vi "P4CMD Dialog - File Properties.vi"(7 "fstat data":string, 8 "error in (no error)":errorcluster, 10 "opened data":string, 11 "source control reference in":T1) -> (0 "error out":errorcluster)   [LabVIEW 2017, in "NI_SCC_P4CMD.lvlib"]
uses:
  <vilib>/SourceControl/Providers/P4CMD/NI_SCC_P4CMD.lvlib
  <vilib>/SourceControl/sccapi/SCCAPI Refnum.ctl
  <vilib>/SourceControl/Providers/P4CMD/P4CMD Operations.ctl
  <vilib>/event_ctls.llb/eventvkey.ctl
  <vilib>/SourceControl/sccapi/NI_SCC.lvlib
panel:
  in  "Describe":bool
  in  "help":bool
  out "locked by":string caption="Locked By:"
  in  "opened by":i32(listbox) caption="Opened For:"
  out "last mode time":string caption="Last ModTime:"
  out "head change":string caption="Head Change:"
  out "have revision":string caption="Have Revision:"
  out "head action":string caption="Head Action:"
  out "head revision":string caption="Head Revision:"
  out "file type":string caption="File Type:"
  out "client path":string caption="Client Path:"
  out "depot path":string caption="Depot Path:"
  in  "ok":bool
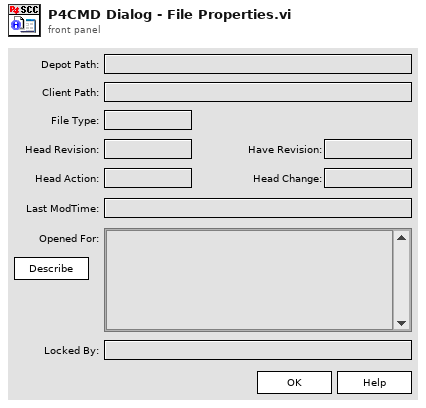
[diagram p1: front panel]
types:
  T1 = typedef "NI_SCC.lvlib/SCCAPI Refnum.ctl" = refnum<k1>
  T2 = typedef "NI_SCC_P4CMD.lvlib/P4CMD Operations.ctl" = enum16{"get all clients", "get all users", "describe changelist", "sync from depot", "open for edit", "submit to depot", "revert", "add to depot", "remove from depot", "print files revisions", "compare client file", "print depot file contents", "list opened files", "get file info", "lock files", "edit changelist spec", "info", "set variables"}
  T3 = typedef "eventvkey.ctl" = enum16{"ASCII", "Enter", "Return", "Shift", "Ctrl", "Alt", "Cmd", "Opt", "Caps", "NumLock", "Clear", "Break", "Up", "Down", "Left", "Right", "Insert", "Delete", "Home", "End", "PageUp", "PageDown", "Escape", "Help", "Pause", "ScrollLock", "F1", "F2", "F3", "F4", "F5", "F6", "F7", "F8", "F9", "F10", "F11", "F12", "F13", "F14", "F15", "F16", "F17", "F18", "F19", "F20", "F21", "F22", "F23", "F24", "Play", "VolumeUp", "VolumeDown", "Mute", "Two Byte Char"}
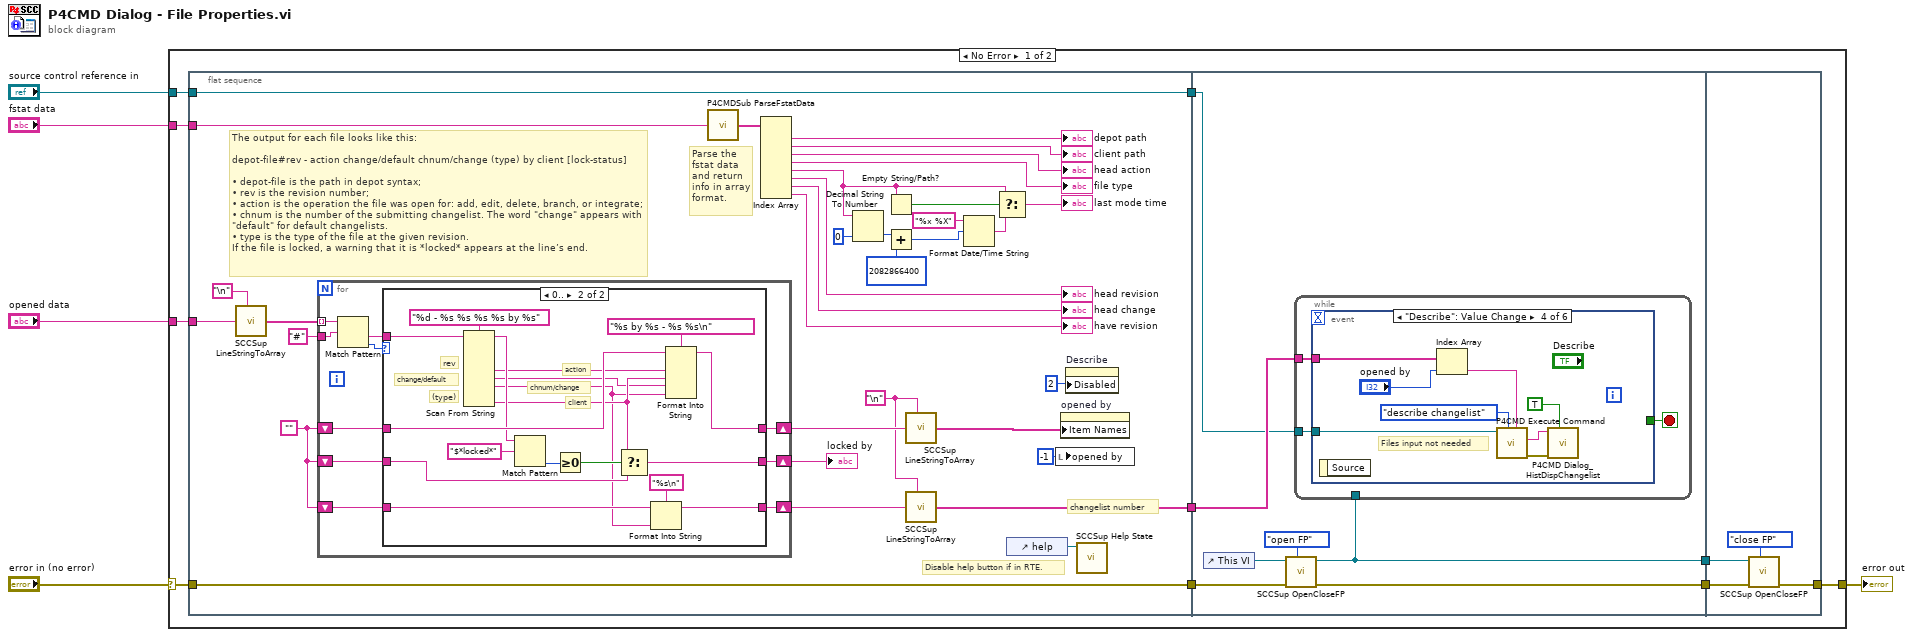
[diagram p0: block diagram]
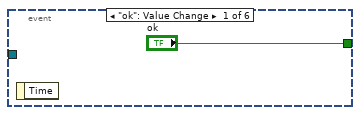
[diagram p3: hidden frame]
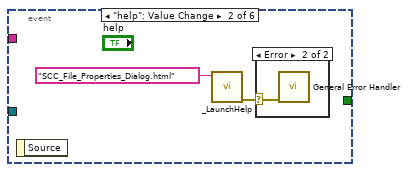
[diagram p4: hidden frame]
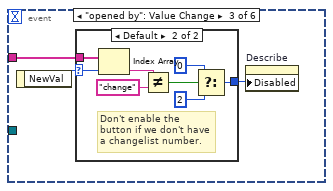
[diagram p6: hidden frame]
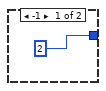
[diagram p7: hidden frame]
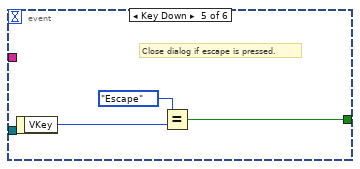
[diagram p8: hidden frame]
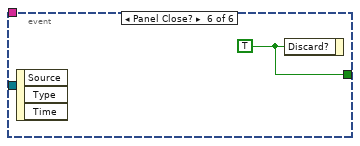
[diagram p9: hidden frame]
diagram:
  n1 = case shown="No Error" "error in (no error)" {
    selector: "error in (no error)" -> [w15 w123]
    tunnel: [w11 w123] -> w4
    tunnel: "fstat data" -> [w10 _]
    tunnel: "opened data" -> [w9 _]
    tunnel: "source control reference in" -> [w7 _]
    frame No Error {
      n2 = flat-sequence {
        tunnel: w15 -> [w49]
        tunnel: [w49] -> w14
        tunnel: w10 -> [w48]
        tunnel: w9 -> [w47]
        tunnel: [w17] -> w8
        tunnel: w7 -> [w16]
        tunnel: [w16] -> w6
        tunnel: w14 -> [w84]
        tunnel: [w87] -> w13
        tunnel: [w86] -> w12
        tunnel: w8 -> [w82]
        tunnel: w6 -> [w81]
        tunnel: w13 -> [w121]
        tunnel: w12 -> [w120]
        tunnel: [w119] -> w11
        frame #0 {
          w19 = "\n" ("Line Feed Constant")
          w24 = "" ("Empty String Constant")
          # "changelist number"
          # "The output for each file looks like this:\n\ndepot-file#rev - action change/default chnum/change (type) by client [lock-status]\n\n• depot-file is the path in depot syntax;\n• rev is the revision number;\n• action is the operation the file was open for: add, edit, delete, branch, or integrate;\n• chnum is the number of the submitting changelist. The word \"change\" appears with \"default\" for default changelists.\n• type is the type of the file at the given revision.\nIf the file is locked, a warning that it is *locked* appears at the line’s end."
          # "Parse the fstat data and return info in array format."
          # "Disable help button if in RTE."
          n3 = call <vilib>:"SCCSup LineStringToArray.vi"("delimiter (Tab)"="\n" ("Line Feed Constant"), "line string"=w47) -> ("line array"=w40:string[])  [unwired: 7 in]
          n4 = for {
            tunnel: w40 -> [w55] mode=indexing
            shift-right: [w56] -> w21
            shift-left: w24 -> [w57]
            shift-right: [w53] -> w32
            shift-left: w24 -> [w54]
            tunnel: "#" ("regular expression") -> [w52]
            shift-right: [w51] -> w18
            shift-left: w24 -> [w50]
            n5 = Match Pattern(string=w55, regular expression=w52) -> (after substring=w58:string, offset past match=w59:i32)  [unwired: 1 in, 2 out]
            n6 = case shown="0.." w59 {
              tunnel: w58 -> [_ w80]
              tunnel: w57 -> [w62 w78]
              tunnel: [w62 w76] -> w56
              tunnel: w54 -> [w61 w70]
              tunnel: [w61 w71] -> w53
              tunnel: [w60 w66] -> w51
              tunnel: w50 -> [w60 w65]
              frame Default {
              }
              frame 0.. {
                # "client"
                # "(type)"
                # "chnum/change"
                # "change/default"
                # "action"
                # "rev"
                n7 = Scan From String(format string="%d - %s %s %s %s by %s" ("Format String"), input string=w80) -> (remaining string=w74:string, output 2=w68:string, output 3=w63:string, output 4=w64:string, output 6=w69:string)  [unwired: 10 in, 2 out]
                n8 = Match Pattern(string=w74, regular expression="$*locked*") -> (offset past match=w72:i32)  [unwired: 1 in, 3 out]
                n9 = Greater Or Equal To 0?(x=w72) -> (x >= 0?=w73:bool)
                n10 = Select(t=w69, s=w73, f=w70) -> (s? t:f=w71:string)
                n11 = Format Into String(format string="%s\n", initial string=w65, w64) -> (resulting string=w66:string)  [unwired: 1 in, 1 out]
                n12 = Format Into String(format string="%s by %s - %s %s\n" ("Format String"), initial string=w78, w68, w69, w63, w64) -> (resulting string=w76:string)  [unwired: 1 in, 1 out]
              }
            }
          }
          "locked by" <- w32
          n13 = call <vilib>:"P4CMDSub ParseFstatData.vi"("fstat data"=w48) -> ("parsed array"=w46:string[])  [unwired: 4 in]
          n14 = Index Array(array=w46) -> (element #1=→"depot path":string, element #2=→"client path":string, element #3=→"head action":string, element #4=→"file type":string, element #5=w28:string, element #6=→"head revision":string, element #7=→"head change":string, element #8=→"have revision":string)  [unwired: 8 in]
          n15 = Decimal String To Number(string=w28, default (0L)=u32 0) -> (number=w45:u32)  [unwired: 1 in, 1 out]
          n16 = Empty String/Path?(string/path=w28) -> (empty?=w31:bool)
          n17 = Add(x=w45, y=u32 2082866400 ("seconds")) -> (x+y=w41:u32)
          n18 = call <vilib>:"SCCSup LineStringToArray.vi"("delimiter (Tab)"=w19, "line string"=w21) -> ("line array"=w20:string[])  [unwired: 7 in]
          n19 = call <vilib>:"SCCSup LineStringToArray.vi"("delimiter (Tab)"=w19, "line string"=w18) -> ("line array"=w17:string[])  [unwired: 7 in]
          n20 = Format Date/Time String(time format string (%c)="%x %X", seconds (now)=w41) -> (date/time string=w29:string)  [unwired: 1 in]
          n21 = Select(t=w28, s=w31, f=w29) -> (s? t:f=→"last mode time":string)
          n22 = control-ref of="help"() -> (w25:refnum<vi>)
          n23 = local write "opened by"(-1 ("opened by")) -> ()
          n24 = property on="opened by" class="LstBox (strict)"("Item Names"=w20) -> ()  [unwired: 2 in, 2 out]
          n25 = property on="Describe" class="Bool"("Disabled"=u8 2) -> ()  [unwired: 2 in, 2 out]
          n26 = call <vilib>:"SCCSup Help State.vi"("help ref"=w25) -> ()  [unwired: 10 in, 1 out]
        }
        frame #1 {
          n27 = control-ref of="This VI"() -> (w83:refnum<vi>)
          n28 = call <vilib>:"SCCSup OpenCloseFP.vi"("function"=enum16{"open FP", "close FP"}."open FP", "error in (no error)"=w84, "VI Refnum in"=w83) -> ("error out"=w86:errorcluster, "VI Refnum out"=w87:refnum<vi>)  [unwired: 7 in]
          n29 = while {
            tunnel: w87 -> [_]
            tunnel: w82 -> [w89]
            tunnel: w81 -> [w88]
            stop <- w90 stop-if-true
            n30 = event shown="[3] \"Describe\": Value Change" {
              selector: _ -> [_ _ _ _ _ _]
              dyn-events: _ -> [_ _ _ _ _ _]
              timeout: _ -> [_ _ _ _ _ _]
              tunnel: ["ok" _ _ _ w115 w118] -> w90
              tunnel: w89 -> [_ _ w97 w110 _ _]
              tunnel: w88 -> [_ _ _ w107 _ _]
              event "ok": Value Change {
                n31 = event-data() -> ()  [unwired: 1 in, 1 out]
              }
              event "help": Value Change {
                n32 = event-data() -> ()  [unwired: 1 in, 1 out]
                n33 = call <helpdir>:"_LaunchHelp.vi"("HTML filename"="SCC_File_Properties_Dialog.html" ("Help topic")) -> ("error out"=w93:errorcluster)  [unwired: 6 in]
                n34 = case shown="Error" w93 {
                  selector: w93 -> [_ w94]
                  frame No Error {
                  }
                  frame Error {
                    n35 = call <vilib>:"General Error Handler.vi"("error in (no error)"=w94) -> ()  [unwired: 10 in, 5 out]
                  }
                }
              }
              event "opened by": Value Change {
                n36 = event-data() -> ("NewVal"=w95:i32)  [unwired: 1 in]
                n37 = case shown="Default" w95 {
                  selector: w95 -> [_ w100]
                  tunnel: w97 -> [_ w106]
                  tunnel: [u8 2 ("Disabled") w99] -> w96
                  frame -1 {
                  }
                  frame Default {
                    # "Don't enable the button if we don't have a changelist number."
                    n38 = Index Array(array=w106, index=w100) -> (element=w105:string)
                    n39 = Not Equal?(x=w105, y="change") -> (x != y?=w103:bool)
                    n40 = Select(t=u8 0 ("Disabled"), s=w103, f=u8 2 ("Disabled")) -> (s? t:f=w99:u8)
                  }
                }
                n41 = property on="Describe" class="Bool"("Disabled"=w96) -> ()  [unwired: 2 in, 2 out]
              }
              event "Describe": Value Change {
                # "Files input not needed"
                n42 = event-data() -> ()  [unwired: 1 in, 1 out]
                n43 = Index Array(array=w110, index="opened by") -> (element=w114:string)
                n44 = call <vilib>:"P4CMD Execute Command.vi"("optional operation parameters"=w114, "p4 operation"=P4CMD_Operations."describe changelist", "source control reference in"=w107) -> ("error out"=w111:errorcluster, "command information"=w112:string)  [unwired: 6 in, 1 out]
                n45 = call <vilib>:"P4CMD Dialog_HistDispChangelist.vi"("Hide diff checkbox?"=TRUE, "error in (no error)"=w111, "changelist description"=w112) -> ()  [unwired: 8 in, 1 out]
              }
              event Key Down {
                # "Close dialog if escape is pressed."
                n46 = event-data() -> ("VKey"=w117:T3)  [unwired: 1 in]
                n47 = Equal?(x=eventvkey."Escape", y=w117) -> (x = y?=w115:bool)
              }
              event Panel Close? {
                w118 = TRUE ("Discard?")
                n48 = event-data() -> ()  [unwired: 1 in, 3 out]
                n49 = event-data ("Event Filter Node")("Discard?"=w118) -> ()  [unwired: 1 in, 1 out]
              }
            }
          }
        }
        frame #2 {
          n50 = call <vilib>:"SCCSup OpenCloseFP.vi"("function"=enum16{"open FP", "close FP"}."close FP", "error in (no error)"=w120, "VI Refnum in"=w121) -> ("error out"=w119:errorcluster)  [unwired: 7 in, 1 out]
        }
      }
    }
    frame Error {
    }
  }
  "error out" <- w4
